vi "Stop Core.vi"(10 "final error code":i32, 11 "AirMar150WX in":refnum<class "AirMar150WX.lvclass">) -> (3 "AirMar150WX out":refnum<class "AirMar150WX.lvclass">)   [LabVIEW 2017, in "AirMar 150WX.lvlib" / "AirMar150WX.lvclass"]
doc: "In addition to the following, this method also sends a message to the monitor to notify it that the actor has stopped execution.\n\n(<B>Filename</B>: Actor Framework.lvlib:Actor.lvclass:Stop Core.vi)\n\nDefines what the actor does before it stops. Use the <B>final error code</B> input to determine whether the actor shut down in response to an error.\n\nBy default, this method does nothing. A descendant class may override it to define behavior, such as shutting down any processes the actor initiated in its override of the Actor Core method.\n\nCopyright: MGI\nAuthored by: Derek Trepanier"
uses:
  AirMar150WX.lvclass
  AirMar150WX.lvclass/AirMar150WX.ctl
  Sensor Actor/Sensor/Sensor.lvclass
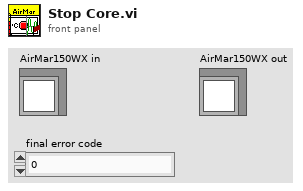
[diagram p1: front panel]
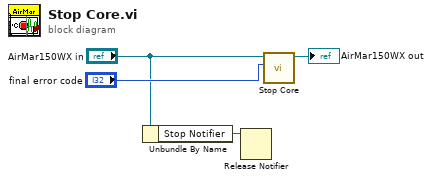
[diagram p0: block diagram]
diagram:
  n1 = Unbundle By Name("AirMar150WX in") -> ("Stop Notifier"=w1:refnum<notifier>)
  n2 = Release Notifier(notifier=w1) -> ()  [unwired: 2 in, 3 out]
  n3 = call-parent "Stop Core.vi"("final error code"="final error code", "Sensor in"="AirMar150WX in") -> ("Sensor out"=→"AirMar150WX out":refnum<class "AirMar150WX.lvclass">)  [unwired: 9 in]
